vi "Init Resistive Sim page.vi"(6 "Resistive sim controls":refnum<vi>[](array[refnum]), 7 "Card Position":refnum<vi>, 8 "error in (no error)":errorcluster, 9 "Description":refnum<vi>, 10 "Name":refnum<vi>, 11 "Node Ptr":T1 format="%.0x") -> (0 "error out":errorcluster, 3 "Node Ptr out":T1 format="%.0x")   [LabVIEW 2014, in "SLSC configuration System Explorer.lvlib"]
uses:
  SLSC configuration System Explorer.lvlib
  <vilib>/NI Veristand/Custom Device API/Custom Device Item Ref.ctl
  Shared/Card Postion.ctl
  Shared/Constants.vi
  <vilib>/NI Veristand/Custom Device API/Get Item Property (Variant).vi
  <vilib>/NI Veristand/Custom Device API/Get Item Property (U16).vi
  <vilib>/NI Veristand/Custom Device API/Custom Device API.lvlib
  Shared/SLSC configuration Shared.lvlib
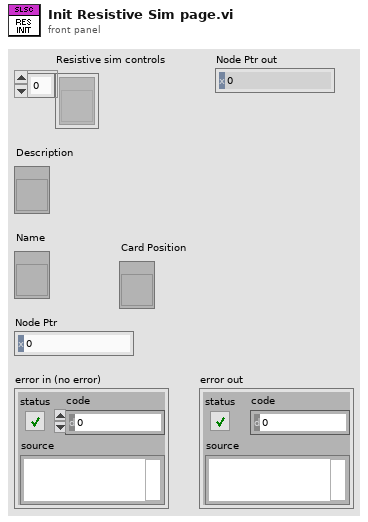
[diagram p1: front panel]
types:
  T1 = typedef "Custom Device API.lvlib/Custom Device Item Ref.ctl" = u64
  T2 = typedef "SLSC configuration Shared.lvlib/Card Postion.ctl" = cluster{"Chassis #":u8, "Slot #":u8}
  T3 = typedef "Custom Device API.lvlib/Custom Device Item Info.ctl" = cluster{"Name":string, "Is Channel":bool, "GUID":string, "Is Waveform":bool}
  T4 = typedef "Custom Device API.lvlib/Custom Device Channel.ctl" = cluster{"Type":T5, "Units":string, "Default Value":dbl, "Faultable":bool, "Scalable":bool}
  T5 = typedef "Custom Device API.lvlib/Custom Device Channel Type.ctl" = enum16{"Input", "Output"}
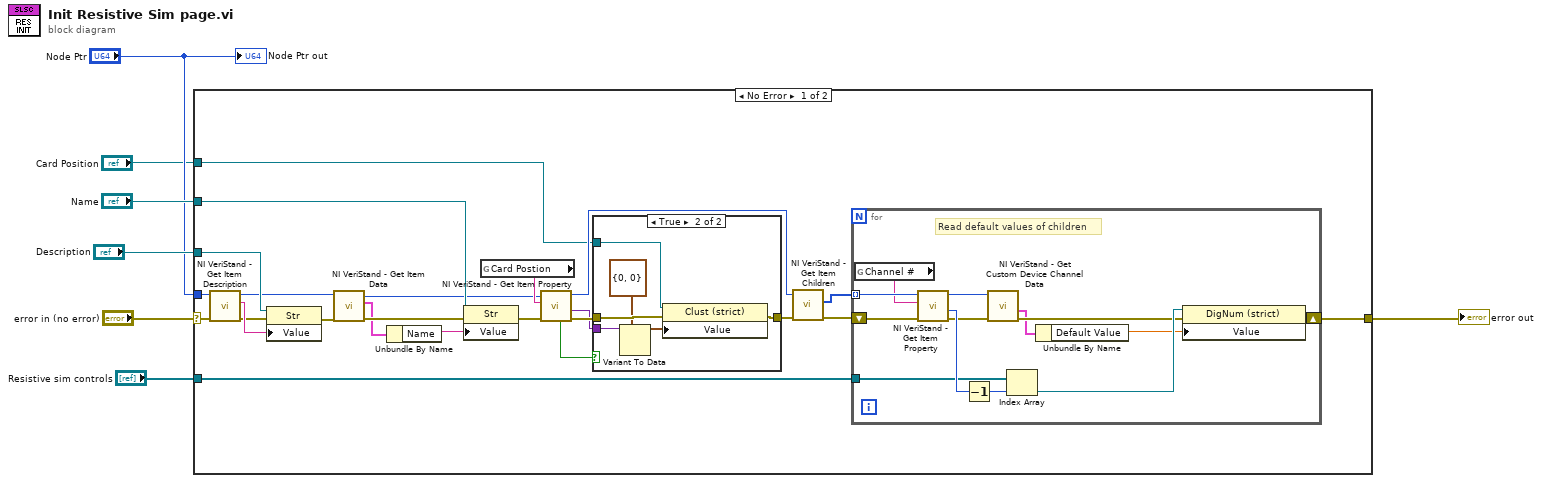
[diagram p0: block diagram]
diagram:
  n1 = case shown="No Error" "error in (no error)" {
    selector: "error in (no error)" -> [w14 w52]
    tunnel: "Name" -> [w31 _]
    tunnel: "Description" -> [w27 _]
    tunnel: "Resistive sim controls" -> [w21 _]
    tunnel: [w20 w52] -> w4
    tunnel: "Node Ptr" -> [w19 _]
    tunnel: "Card Position" -> [w9 _]
    frame No Error {
      n2 = call <vilib>:"NI VeriStand - Get Item Description.vi"("error in (no error)"=w14, "Item Ref in"=w19) -> ("error out"=w26:errorcluster, "Description"=w28:string, "Item Ref out"=w22:T1)  [unwired: 7 out]
      n3 = property class="Str"(reference=w27, error in=w26, "Value"=w28) -> (error out=w29:errorcluster)  [unwired: 1 out]
      n4 = call <vilib>:"NI VeriStand - Get Item Data.vi"("error in (no error)"=w29, "Item Ref in"=w22) -> ("error out"=w30:errorcluster, "Item Info"=w23:T3, "Item Ref out"=w15:T1)  [unwired: 7 out]
      n5 = Unbundle By Name(w23) -> ("Name"=w8:string)
      n6 = property class="Str"(reference=w31, error in=w30, "Value"=w8) -> (error out=w17:errorcluster)  [unwired: 1 out]
      n7 = global read "Constants.vi" "Card Postion"() -> (w18:string)
      n8 = call-poly <vilib>:"NI VeriStand - Get Item Property.vi"("error in (no error)"=w17, "Property Name"=w18, "Item Ref in"=w15) -> ("error out"=w11:errorcluster, "Value"=w10:variant, "Item Ref out"=w16:T1, "Found?"=w12:bool)  [unwired: 5 in]
      n9 = case shown="True" w12 {
        tunnel: w11 -> [w32 w38]
        tunnel: [w32 w37] -> w13
        tunnel: w10 -> [_ w36]
        tunnel: w9 -> [_ w33]
        frame False {
        }
        frame True {
          n10 = Variant To Data(type=T2 {"Chassis #"=0, "Slot #"=0} ("Card Position"), Variant=w36) -> (data=w35:T2)  [unwired: 1 in, 1 out]
          n11 = property class="Clust (strict)"(reference=w33, error in=w38, "Value"=w35) -> (error out=w37:errorcluster)  [unwired: 1 out]
        }
      }
      n12 = call <vilib>:"NI VeriStand - Get Item Children.vi"("error in (no error)"=w13, "Item Ref in"=w16) -> ("error out"=w24:errorcluster, "Child Refs"=w25:T1[])  [unwired: 6 in, 2 out]
      n13 = for {
        tunnel: w25 -> [w51] mode=indexing
        tunnel: w21 -> [w47]
        shift-right: [w43] -> w20
        shift-left: w24 -> [w49]
        # "Read default values of children"
        n14 = global read "Constants.vi" "Channel #"() -> (w50:string)
        n15 = call-poly <vilib>:"NI VeriStand - Get Item Property.vi"("error in (no error)"=w49, "Property Name"=w50, "Item Ref in"=w51) -> ("error out"=w42:errorcluster, "Value"=w48:u16, "Item Ref out"=w44:T1)  [unwired: 5 in, 1 out]
        n16 = Decrement(x=w48) -> (x-1=w46:u16)
        n17 = call <vilib>:"NI VeriStand - Get Custom Device Channel Data.vi"("error in (no error)"=w42, "Channel Ref in"=w44) -> ("error out"=w41:errorcluster, "Channel"=w40:T4)  [unwired: 4 in, 4 out]
        n18 = Index Array(array=w47, index=w46) -> (element=w45:refnum<vi>)
        n19 = Unbundle By Name(w40) -> ("Default Value"=w39:dbl)
        n20 = property class="DigNum (strict)"(reference=w45, error in=w41, "Value"=w39) -> (error out=w43:errorcluster)  [unwired: 1 out]
      }
    }
    frame Error {
    }
  }
  "error out" <- w4
  "Node Ptr out" <- "Node Ptr"
